vi "sonar task.vi"(11 "AIDeviceRef":T1) -> ()   [LabVIEW 2011]
uses:
  <vilib>/Rock Robotics/WPI/AnalogChannel/WPI_AnalogChannelDevRef.ctl
  <vilib>/Rock Robotics/SystemInterfaces/Typedef/FPGA_TypedefAnalogModule.ctl
  <vilib>/Rock Robotics/SystemInterfaces/AI/FPGA_AIChannel.ctl
  Robot Global Data.vi
panel:
  out "Voltage":dbl
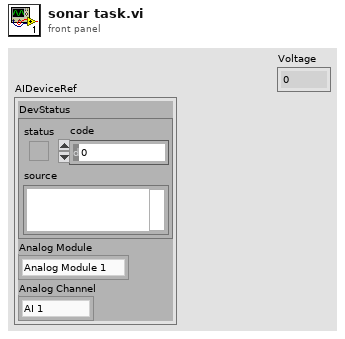
[diagram p1: front panel]
types:
  T1 = typedef "WPI_AnalogChannelDevRef.ctl" = cluster{"DevStatus":errorcluster, "Analog Module":T2, "Analog Channel":T3}
  T2 = typedef "FPGA_TypedefAnalogModule.ctl" = enum16{"Analog Module 1", "Analog Module 2"}
  T3 = typedef "FPGA_AIChannel.ctl" = enum8{"AI 1", "AI 2", "AI 3", "AI 4", "AI 5", "AI 6", "AI 7", "AI 8", "Invalid"}
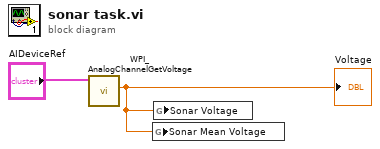
[diagram p0: block diagram]
diagram:
  n1 = call <vilib>:"WPI_AnalogChannelGetVoltage.vi"("AIDeviceRef"="AIDeviceRef") -> ("Voltage"=w1:dbl)  [unwired: 8 in, 2 out]
  "Voltage" <- w1
  n2 = global write "Robot Global Data.vi" "Sonar Mean Voltage"(w1) -> ()
  n3 = global write "Robot Global Data.vi" "Sonar Voltage"(w1) -> ()
